vi "Analyze Data.vi"(8 "error in":errorcluster, 11 "nCRD in":refnum<class "gCRD.lvclass">) -> (0 "error out":errorcluster, 3 "nCRD out":refnum<class "gCRD.lvclass">)   [LabVIEW 2017, in "gCRDS.lvlib" / "gCRD.lvclass"]
doc: "Analyze Data takes the stored ringdown data (1000 shots per cell) and:\n1) Calculates the ringdown decay constant tau\n2) Averages tau0 data as necessary\n3) Corrects the tau data for Rayleigh scattering\n4) Stores a 1-D array of taus returned on a 1 kHz basis (8k taus) if a jump drive (U:) is connected\n5) Flattens the data into a string and stuffs the string into the <b>data</b> shared variable for display on the UI.\n\nThis VI will not be called if the data is not \"good\" (that is, if an error was thrown in the <B>Get Data</B> routine. If an error is thrown while the data is being retrieved, then the data will not be sent to the UI."
uses:
  gCRD.lvclass
  C:/Program Files (x86)/National Instruments/LabVIEW 2017/vi.lib/MSR Consulting, LLC/General Reuse/Instrument/Instrument.lvclass
  <vilib>/MSR Consulting, LLC/General Reuse/CRDS/Data/Main/CRDS Data.lvclass
  C:/Program Files (x86)/National Instruments/LabVIEW 2017/vi.lib/MSR Consulting, LLC/General Reuse/Data/Data.lvclass
  <vilib>/MSR Consulting, LLC/General Reuse/CRDS/Data/Cell/CRDS Cell Data.lvclass
  <vilib>/MSR Consulting, LLC/General Reuse/Instrument/Instrument.lvclass/Instrument.ctl
  <vilib>/MSR Consulting, LLC/General Reuse/CRDS/Data/Cell/CRDS Cell Data.lvclass/CRDS Cell Data.ctl
  <vilib>/MSR Consulting, LLC/General Reuse/CRDS/Data/Cell/Write Write RD_.vi
  <vilib>/MSR Consulting, LLC/General Reuse/Instrument/Read Data Notifier.vi
  <vilib>/MSR Consulting, LLC/General Reuse/Instrument/Read Data.vi
  <vilib>/MSR Consulting, LLC/General Reuse/CRDS/Data/Main/Read CellData.vi
  <vilib>/MSR Consulting, LLC/General Reuse/CRDS/Data/Main/Write CellData.vi
  <vilib>/MSR Consulting, LLC/General Reuse/CRDS/Main/CRDS.lvclass
  <vilib>/MSR Consulting, LLC/General Reuse/Data/Data.lvclass
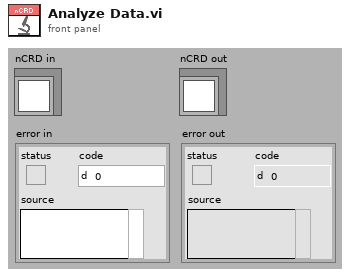
[diagram p1: front panel]
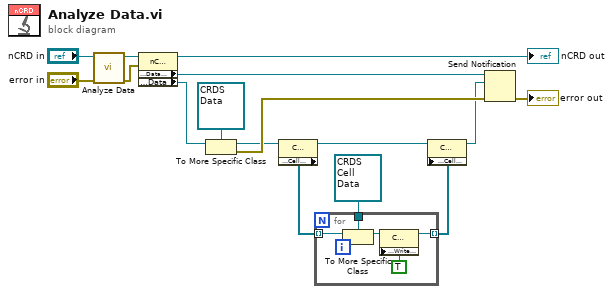
[diagram p0: block diagram]
diagram:
  n1 = call-parent "Analyze Data.vi"("error in"="error in", "CRDS in"="nCRD in") -> ("error out"=w11:errorcluster, "CRDS out"=w12:refnum<class "gCRD.lvclass">)  [unwired: 8 in]
  n2 = property class="nCRD"(reference=w12, error in=w11) -> (reference out=→"nCRD out":refnum<class "gCRD.lvclass">, "Accessors:Data Notifier"=w8:refnum<notifier>, "Accessors:Data"=w9:refnum<class "Data.lvclass">)  [unwired: 1 out]
  n3 = To More Specific Class(target class=refnum<class "CRDS Data.lvclass"> refnum ("CRDS Lib.lvlib:CRDS"), reference=w9) -> (specific class reference=w6:refnum<class "CRDS Data.lvclass">, error out=w7:errorcluster)  [unwired: 1 in]
  n4 = property class="CRDS"(reference=w6) -> (reference out=w3:refnum<class "CRDS Data.lvclass">, "Accessors:Cell Data"=w5:refnum<class "CRDS Cell Data.lvclass">[])  [unwired: 1 in, 1 out]
  n5 = for {
    tunnel: w5 -> [w21] mode=indexing
    tunnel: refnum<class "CRDS Cell Data.lvclass"> refnum ("CRDS Lib.lvlib:CRDS Cell") -> [w19]
    tunnel: [w17] -> w2 mode=indexing
    n6 = To More Specific Class(target class=w19, reference=w21) -> (specific class reference=w20:refnum<class "CRDS Cell Data.lvclass">)  [unwired: 1 in, 1 out]
    n7 = property class="CRDS Cell"(reference=w20, "Data Access:Write RD_"=TRUE ("Write RD_")) -> (reference out=w17:refnum<class "CRDS Cell Data.lvclass">)  [unwired: 1 in, 1 out]
  }
  n8 = property class="CRDS"(reference=w3, "Accessors:Cell Data"=w2) -> (reference out=w1:refnum<class "CRDS Data.lvclass">)  [unwired: 1 in, 1 out]
  n9 = Send Notification(notification=w1, notifier=w8, error in (no error)=w7) -> (error out=→"error out":errorcluster)  [unwired: 1 out]
